vi "CRYInit Curve Library.vi"   [LabVIEW 2013]
uses:
  CRYSystem/Typedef Control/CRYData Cluster.ctl
  CRYSystem/Typedef Control/CRYResult Cluster.ctl
  CRYSystem/Typedef Control/CRYWaveform Cluster.ctl
  Global/CRYCurve Library Global.vi
  CRYMainGlobal.vi
  <vilib>/picture/picture.llb/imagedata.ctl
panel:
  # "Initialize Curve Library global variable"
types:
  T1 = cluster{"Curve OrgNames":string[], "Value OrgNames":string[], "Result OrgNames":string[], "WFM OrgNames":string[], "Curve NewNames":string[], "Value NewNames":string[], "Result NewNames":string[], "WFM NewNames":string[]}
  T2 = typedef "CRYWaveform Cluster.ctl" = cluster{"Waveform":cluster{"X0":dbl, "dX":dbl, "Y":sgl[]}, "X data":u16, "Y data":u16, "Y axis":u16, "X unit":string, "Y unit":string, "Y dB ref":dbl, "display Y":bool, "display X":bool, "Overload?":bool, "Test Info":string, "Step No.":i32, "Name":string, "protected":bool, "Sqc history":string[], "Signal Channel ID":i32, "Plot Settings":cluster{"Color":u32, "Interpolation":u8, "Point Style":u8, "Line Style":u8, "Point Color":u32, "Line Width":u8, "Bar Plot Style":u8, "Fill To":i16}, "AutoProtect":bool}
  T3 = typedef "CRYResult Cluster.ctl" = cluster{"Name":string, "Margin":dbl, "unit":string, "Verdict":bool, "Limit":string, "Max/Min":string, "protected":bool, "Step No.":i32, "Test Info":string, "AutoProtect":bool}
  T4 = cluster{"Type Name":string, "Data Name":string, "Probe VIRef Number":i32, "Probe VIRef":refnum<vi>}[]
  T5 = typedef "imagedata.ctl" = cluster{"image type":i32, "image depth":i32, "image":u8[], "mask":u8[], "colors":u32[], "Rectangle":cluster{"left":i16, "top":i16, "right":i16, "bottom":i16}}
  T6 = cluster{"Left Cell String":string, "Child Text":string[], "Child Tag":string, "Item Indent":i32, "Child Only?":bool, "Glyph Index":i32}[]
  T7 = typedef "CRYData Cluster.ctl" = cluster{"Name":string, "Curve":cluster{"x":dbl, "y":dbl, "z":dbl}[], "X data":u16, "Y data":u16, "Z data":u16, "X axis":u16, "Y axis":u16, "Z axis":u16, "X unit":string, "Y unit":string, "Z unit":string, "X dB ref":dbl, "Y dB ref":dbl, "Z dB ref":dbl, "single val":bool, "protected":bool, "display X":bool, "display Y":bool, "display Z":bool, "Test Info":string, "Step No.":i32, "Plot Settings":cluster{"Color":u32, "Interpolation":u8, "Point Style":u8, "Line Style":u8, "Point Color":u32, "Line Width":u8, "Bar Plot Style":u8, "Fill To":i16}, "AutoProtect":bool}
  T8 = typedef "CRYImageData.ctl" = cluster{"image type":i32, "image depth":i32, "image":u8[], "mask":u8[], "colors":u32[], "Rectangle":cluster{"left":i16, "top":i16, "right":i16, "bottom":i16}}
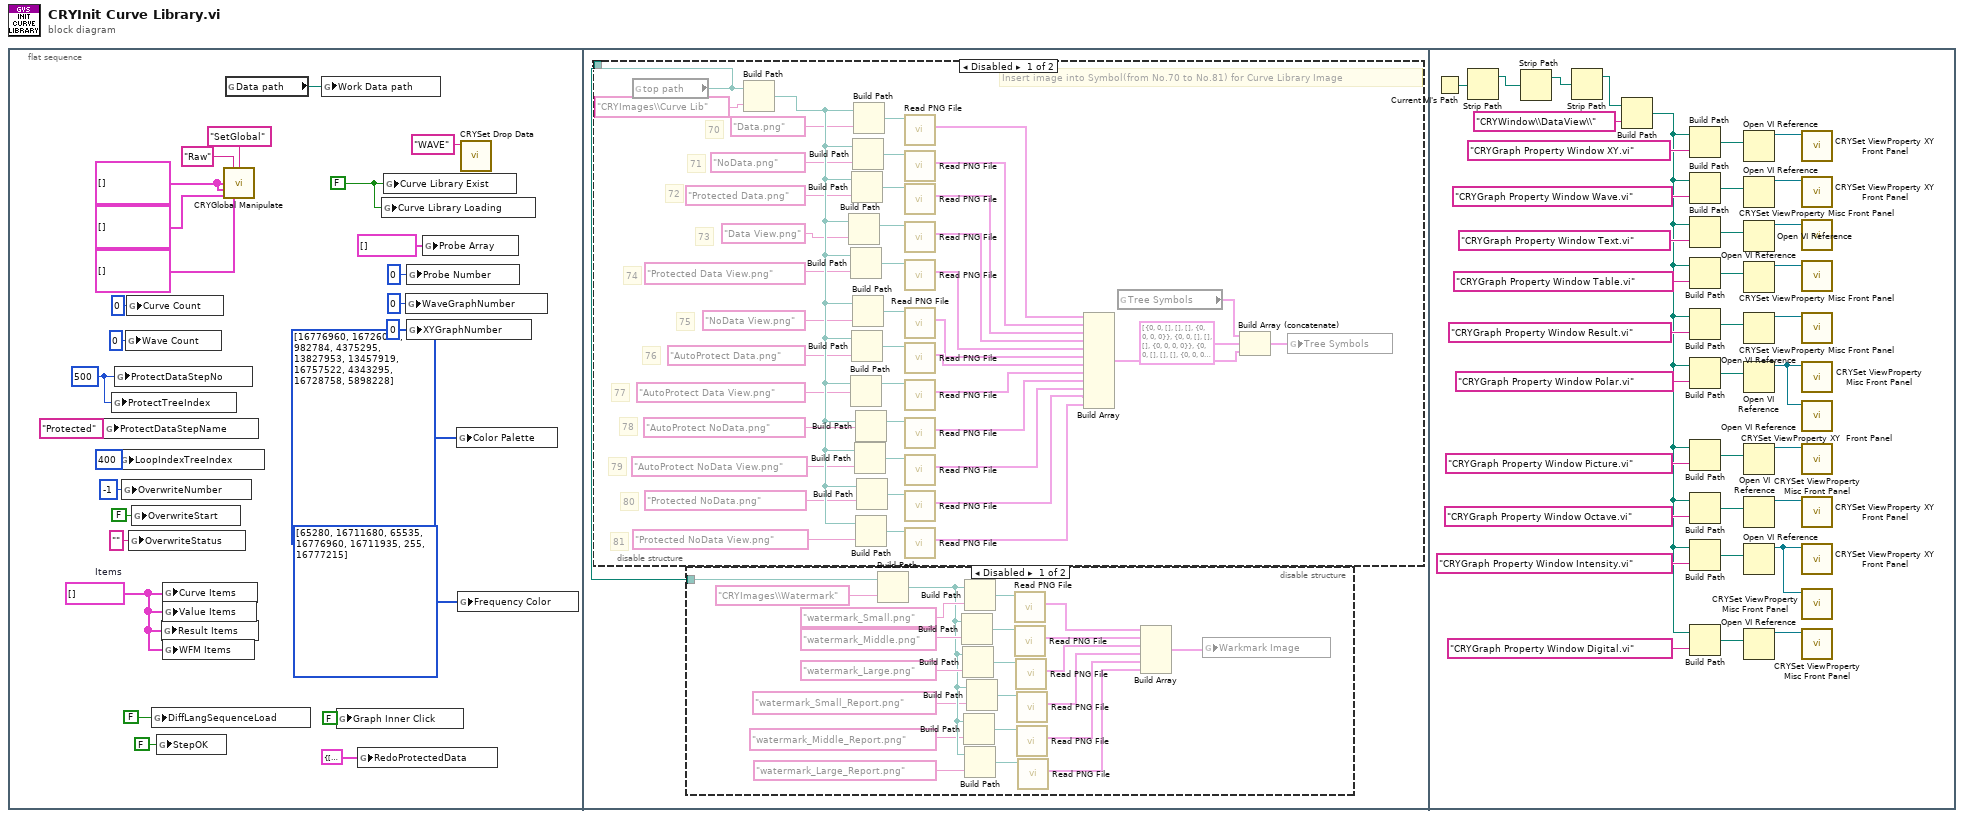
[diagram p0: block diagram]
diagram:
  n1 = flat-sequence {
    frame #0 {
      w6 = 500 ("ProtectStepNo")
      w11 = T6 []  # Items
      w14 = T7[] [] ("Curves")
      w25 = FALSE ("Exist")
      n2 = global write "CRYCurve Library Global.vi" "ProtectDataStepName"("Protected" ("ProtectDataStepName")) -> ()
      n3 = global write "CRYCurve Library Global.vi" "ProtectTreeIndex"(w6) -> ()
      n4 = global write "CRYCurve Library Global.vi" "ProtectDataStepNo"(w6) -> ()
      n5 = global write "CRYCurve Library Global.vi" "LoopIndexTreeIndex"(400 ("ProtectStepNo")) -> ()
      n6 = global write "CRYCurve Library Global.vi" "OverwriteNumber"(-1 ("ProtectStepNo")) -> ()
      n7 = global write "CRYCurve Library Global.vi" "Wave Count"(0 ("Curve Count")) -> ()
      n8 = global write "CRYCurve Library Global.vi" "Curve Count"(0 ("Curve Count")) -> ()
      n9 = global write "CRYCurve Library Global.vi" "OverwriteStatus"("" ("OverwriteStatus")) -> ()
      n10 = global write "CRYCurve Library Global.vi" "OverwriteStart"(FALSE ("OverwriteStart")) -> ()
      n11 = global write "CRYCurve Library Global.vi" "DiffLangSequenceLoad"(FALSE ("SequenceLoad")) -> ()
      n12 = global write "CRYCurve Library Global.vi" "StepOK"(FALSE ("StepOK")) -> ()
      n13 = global write "CRYCurve Library Global.vi" "Result Items"(w11) -> ()
      n14 = global write "CRYCurve Library Global.vi" "Curve Items"(w11) -> ()
      n15 = global write "CRYCurve Library Global.vi" "Value Items"(w11) -> ()
      n16 = global write "CRYCurve Library Global.vi" "WFM Items"(w11) -> ()
      n17 = call "CRYGlobal Manipulate.vi"("sOption"="Raw", "sAction"="SetGlobal", "Curves"=w14, "Values"=w14, "Results"=T3[] [], "WFM"=T2[] []) -> ()  [unwired: 3 in, 7 out]
      n18 = global read "CRYMainGlobal.vi" "Data path"() -> (w2:path)
      n19 = global write "CRYCurve Library Global.vi" "Work Data path"(w2) -> ()
      n20 = global write "CRYCurve Library Global.vi" "Graph Inner Click"(FALSE ("Graph Inner Click")) -> ()
      n21 = global write "CRYCurve Library Global.vi" "RedoProtectedData"(T1 {"Curve OrgNames"=[], "Value OrgNames"=[], "Result OrgNames"=[], "WFM OrgNames"=[], "Curve NewNames"=[], "Value NewNames"=[], "Result NewNames"=[], "WFM NewNames"=[]} ("RedoProtectedData")) -> ()
      n22 = global write "CRYCurve Library Global.vi" "Curve Library Loading"(w25) -> ()
      n23 = global write "CRYCurve Library Global.vi" "Curve Library Exist"(w25) -> ()
      n24 = global write "CRYCurve Library Global.vi" "WaveGraphNumber"(u32 0 ("WaveGraphNumber")) -> ()
      n25 = global write "CRYCurve Library Global.vi" "Probe Number"(0 ("Probe Number")) -> ()
      n26 = global write "CRYCurve Library Global.vi" "XYGraphNumber"(u32 0 ("WaveGraphNumber")) -> ()
      n27 = global write "CRYCurve Library Global.vi" "Probe Array"(T4 [] ("Probe Array")) -> ()
      n28 = global write "CRYCurve Library Global.vi" "Color Palette"(u32[] [16776960, 16726034, 982784, 4375295, 13827953, 13457919, 16757522, 4343295, 16728758, 5898228] ("Color Palette")) -> ()
      n29 = global write "CRYCurve Library Global.vi" "Frequency Color"(u32[] [65280, 16711680, 65535, 16776960, 16711935, 255, 16777215] ("Color Palette")) -> ()
      n30 = call "CRYSet Drop Data.vi"("Graph Type In"="WAVE" ("DataType In")) -> ()  [unwired: 11 out]
    }
    frame #1 {
      n31 = disable-structure shown="Disabled" {
        disable-tunnel: [w29 _] -> w28
        frame Disabled {
          # "Insert image into Symbol(from No.70 to No.81) for Curve Library Image"
          # "80"
          # "79"
          # "78"
          # "81"
          # "77"
          # "76"
          # "75"
          # "74"
          # "73"
          # "72"
          # "71"
          # "70"
          n32 = global read "CRYMainGlobal.vi" "top path"() -> (w29:path)
          n33 = Build Path(base path=w29, name or relative path="CRYImages\\Curve Lib") -> (appended path=w70:path)
          n34 = Build Path(base path=w70, name or relative path="Data View.png") -> (appended path=w35:path)
          n35 = Build Path(base path=w70, name or relative path="Protected Data View.png") -> (appended path=w34:path)
          n36 = Build Path(base path=w70, name or relative path="AutoProtect Data View.png") -> (appended path=w42:path)
          n37 = Build Path(base path=w70, name or relative path="Protected Data.png") -> (appended path=w36:path)
          n38 = Build Path(base path=w70, name or relative path="AutoProtect Data.png") -> (appended path=w41:path)
          n39 = Build Path(base path=w70, name or relative path="NoData.png") -> (appended path=w37:path)
          n40 = Build Path(base path=w70, name or relative path="NoData View.png") -> (appended path=w30:path)
          n41 = Build Path(base path=w70, name or relative path="Data.png") -> (appended path=w39:path)
          n42 = Build Path(base path=w70, name or relative path="AutoProtect NoData View.png") -> (appended path=w45:path)
          n43 = Build Path(base path=w70, name or relative path="AutoProtect NoData.png") -> (appended path=w46:path)
          n44 = Build Path(base path=w70, name or relative path="Protected NoData View.png") -> (appended path=w54:path)
          n45 = Build Path(base path=w70, name or relative path="Protected NoData.png") -> (appended path=w53:path)
          n46 = call <vilib>:"Read PNG File.vi"("path to PNG file"=w39) -> ("image data"=w56:T5)  [unwired: 1 in, 9 out]
          n47 = call <vilib>:"Read PNG File.vi"("path to PNG file"=w37) -> ("image data"=w57:T5)  [unwired: 1 in, 9 out]
          n48 = call <vilib>:"Read PNG File.vi"("path to PNG file"=w36) -> ("image data"=w58:T5)  [unwired: 1 in, 9 out]
          n49 = call <vilib>:"Read PNG File.vi"("path to PNG file"=w35) -> ("image data"=w59:T5)  [unwired: 1 in, 9 out]
          n50 = call <vilib>:"Read PNG File.vi"("path to PNG file"=w34) -> ("image data"=w60:T5)  [unwired: 1 in, 9 out]
          n51 = call <vilib>:"Read PNG File.vi"("path to PNG file"=w30) -> ("image data"=w61:T5)  [unwired: 1 in, 9 out]
          n52 = call <vilib>:"Read PNG File.vi"("path to PNG file"=w41) -> ("image data"=w62:T5)  [unwired: 1 in, 9 out]
          n53 = call <vilib>:"Read PNG File.vi"("path to PNG file"=w42) -> ("image data"=w63:T5)  [unwired: 1 in, 9 out]
          n54 = call <vilib>:"Read PNG File.vi"("path to PNG file"=w46) -> ("image data"=w64:T5)  [unwired: 1 in, 9 out]
          n55 = call <vilib>:"Read PNG File.vi"("path to PNG file"=w45) -> ("image data"=w65:T5)  [unwired: 1 in, 9 out]
          n56 = call <vilib>:"Read PNG File.vi"("path to PNG file"=w53) -> ("image data"=w66:T5)  [unwired: 1 in, 9 out]
          n57 = call <vilib>:"Read PNG File.vi"("path to PNG file"=w54) -> ("image data"=w67:T5)  [unwired: 1 in, 9 out]
          n58 = Build Array(w56, w57, w58, w59, w60, w61, w62, w63, w64, w65, w66, w67) -> (w68:T5[])
          n59 = global read "CRYMainGlobal.vi" "Tree Symbols"() -> (w55:T8[])
          n60 = Build Array (concatenate)(w55, T5[] [{"image type"=0, "image depth"=0, "image"=[], "mask"=[], "colors"=[], "Rectangle"={"left"=0, "top"=0, "right"=0, "bottom"=0}}, {"image type"=0, "image depth"=0, "image"=[], "mask"=[], "colors"=[], "Rectangle"={"left"=0, "top"=0, "right"=0, "bottom"=0}}, {"image type"=0, "image depth"=0, "image"=[], "mask"=[], "colors"=[], "Rectangle"={"left"=0, "top"=0, "right"=0, "bottom"=0}}, {"image type"=0, "image depth"=0, "image"=[], "mask"=[], "colors"=[], "Rectangle"={"left"=0, "top"=0, "right"=0, "bottom"=0}}, {"image type"=0, "image depth"=0, "image"=[], "mask"=[], "colors"=[], "Rectangle"={"left"=0, "top"=0, "right"=0, "bottom"=0}}, {"image type"=0, "image depth"=0, "image"=[], "mask"=[], "colors"=[], "Rectangle"={"left"=0, "top"=0, "right"=0, "bottom"=0}}, {"image type"=0, "image depth"=0, "image"=[], "mask"=[], "colors"=[], "Rectangle"={"left"=0, "top"=0, "right"=0, "bottom"=0}}, {"image type"=0, "image depth"=0, "image"=[], "mask"=[], "colors"=[], "Rectangle"={"left"=0, "top"=0, "right"=0, "bottom"=0}}, {"image type"=0, "image depth"=0, "image"=[], "mask"=[], "colors"=[], "Rectangle"={"left"=0, "top"=0, "right"=0, "bottom"=0}}, {"image type"=0, "image depth"=0, "image"=[], "mask"=[], "colors"=[], "Rectangle"={"left"=0, "top"=0, "right"=0, "bottom"=0}}, {"image type"=0, "image depth"=0, "image"=[], "mask"=[], "colors"=[], "Rectangle"={"left"=0, "top"=0, "right"=0, "bottom"=0}}, {"image type"=0, "image depth"=0, "image"=[], "mask"=[], "colors"=[], "Rectangle"={"left"=0, "top"=0, "right"=0, "bottom"=0}}] ("Array"), w68) -> (w71:T5[])
          n61 = global write "CRYMainGlobal.vi" "Tree Symbols"(w71) -> ()
        }
        frame Enabled {
        }
      }
      n62 = disable-structure shown="Disabled" {
        disable-tunnel: w28 -> [w93 _]
        frame Disabled {
          n63 = Build Path(base path=w93, name or relative path="CRYImages\\Watermark") -> (appended path=w79:path)
          n64 = Build Path(base path=w79, name or relative path="watermark_Middle.png") -> (appended path=w87:path)
          n65 = Build Path(base path=w79, name or relative path="watermark_Large.png") -> (appended path=w86:path)
          n66 = Build Path(base path=w79, name or relative path="watermark_Middle_Report.png") -> (appended path=w80:path)
          n67 = Build Path(base path=w79, name or relative path="watermark_Small.png") -> (appended path=w91:path)
          n68 = Build Path(base path=w79, name or relative path="watermark_Large_Report.png") -> (appended path=w81:path)
          n69 = Build Path(base path=w79, name or relative path="watermark_Small_Report.png") -> (appended path=w78:path)
          n70 = call <vilib>:"Read PNG File.vi"("path to PNG file"=w91) -> ("image data"=w90:T5)  [unwired: 8 in, 2 out]
          n71 = call <vilib>:"Read PNG File.vi"("path to PNG file"=w87) -> ("image data"=w85:T5)  [unwired: 8 in, 2 out]
          n72 = call <vilib>:"Read PNG File.vi"("path to PNG file"=w86) -> ("image data"=w84:T5)  [unwired: 8 in, 2 out]
          n73 = call <vilib>:"Read PNG File.vi"("path to PNG file"=w78) -> ("image data"=w77:T5)  [unwired: 8 in, 2 out]
          n74 = call <vilib>:"Read PNG File.vi"("path to PNG file"=w80) -> ("image data"=w76:T5)  [unwired: 8 in, 2 out]
          n75 = call <vilib>:"Read PNG File.vi"("path to PNG file"=w81) -> ("image data"=w75:T5)  [unwired: 8 in, 2 out]
          n76 = Build Array(w90, w85, w84, w77, w76, w75) -> (w89:T5[])
          n77 = global write "CRYCurve Library Global.vi" "Warkmark Image"(w89) -> ()
        }
        frame Enabled {
        }
      }
    }
    frame #2 {
      n78 = Current VI's Path() -> (path=w97:path)
      n79 = Strip Path(path=w97) -> (stripped path=w96:path)  [unwired: 1 out]
      n80 = Strip Path(path=w96) -> (stripped path=w95:path)  [unwired: 1 out]
      n81 = Strip Path(path=w95) -> (stripped path=w94:path)  [unwired: 1 out]
      n82 = Build Path(base path=w94, name or relative path="CRYWindow\\DataView\\") -> (appended path=w116:path)
      n83 = Build Path(base path=w116, name or relative path="CRYGraph Property Window XY.vi") -> (appended path=w126:path)
      n84 = Build Path(base path=w116, name or relative path="CRYGraph Property Window Wave.vi") -> (appended path=w114:path)
      n85 = Build Path(base path=w116, name or relative path="CRYGraph Property Window Text.vi") -> (appended path=w115:path)
      n86 = Build Path(base path=w116, name or relative path="CRYGraph Property Window Table.vi") -> (appended path=w112:path)
      n87 = Build Path(base path=w116, name or relative path="CRYGraph Property Window Result.vi") -> (appended path=w111:path)
      n88 = Build Path(base path=w116, name or relative path="CRYGraph Property Window Polar.vi") -> (appended path=w110:path)
      n89 = Build Path(base path=w116, name or relative path="CRYGraph Property Window Picture.vi") -> (appended path=w109:path)
      n90 = Build Path(base path=w116, name or relative path="CRYGraph Property Window Octave.vi") -> (appended path=w108:path)
      n91 = Build Path(base path=w116, name or relative path="CRYGraph Property Window Intensity.vi") -> (appended path=w106:path)
      n92 = Build Path(base path=w116, name or relative path="CRYGraph Property Window Digital.vi") -> (appended path=w105:path)
      n93 = Open VI Reference(vi path=w126) -> (vi reference=w128:refnum<vi>)  [unwired: 5 in, 1 out]
      n94 = Open VI Reference(vi path=w114) -> (vi reference=w113:refnum<vi>)  [unwired: 5 in, 1 out]
      n95 = Open VI Reference(vi path=w115) -> (vi reference=w104:refnum<vi>)  [unwired: 5 in, 1 out]
      n96 = Open VI Reference(vi path=w112) -> (vi reference=w103:refnum<vi>)  [unwired: 5 in, 1 out]
      n97 = Open VI Reference(vi path=w111) -> (vi reference=w102:refnum<vi>)  [unwired: 5 in, 1 out]
      n98 = Open VI Reference(vi path=w110) -> (vi reference=w98:refnum<vi>)  [unwired: 5 in, 1 out]
      n99 = Open VI Reference(vi path=w109) -> (vi reference=w101:refnum<vi>)  [unwired: 5 in, 1 out]
      n100 = Open VI Reference(vi path=w108) -> (vi reference=w107:refnum<vi>)  [unwired: 5 in, 1 out]
      n101 = Open VI Reference(vi path=w106) -> (vi reference=w100:refnum<vi>)  [unwired: 5 in, 1 out]
      n102 = Open VI Reference(vi path=w105) -> (vi reference=w99:refnum<vi>)  [unwired: 5 in, 1 out]
      n103 = call "CRYSet ViewProperty XY  Front Panel.vi"("Vi Ref"=w128) -> ()  [unwired: 11 in]
      n104 = call "CRYSet ViewProperty XY  Front Panel.vi"("Vi Ref"=w113) -> ()  [unwired: 11 in]
      n105 = call "CRYSet ViewProperty Misc Front Panel.vi"("Vi Ref"=w104) -> ()  [unwired: 11 in]
      n106 = call "CRYSet ViewProperty Misc Front Panel.vi"("Vi Ref"=w103) -> ()  [unwired: 11 in]
      n107 = call "CRYSet ViewProperty Misc Front Panel.vi"("Vi Ref"=w102) -> ()  [unwired: 11 in]
      n108 = call "CRYSet ViewProperty Misc Front Panel.vi"("Vi Ref"=w98) -> ()  [unwired: 11 in]
      n109 = call "CRYSet ViewProperty XY  Front Panel.vi"("Vi Ref"=w98) -> ()  [unwired: 11 in]
      n110 = call "CRYSet ViewProperty Misc Front Panel.vi"("Vi Ref"=w101) -> ()  [unwired: 11 in]
      n111 = call "CRYSet ViewProperty XY  Front Panel.vi"("Vi Ref"=w107) -> ()  [unwired: 11 in]
      n112 = call "CRYSet ViewProperty XY  Front Panel.vi"("Vi Ref"=w100) -> ()  [unwired: 11 in]
      n113 = call "CRYSet ViewProperty Misc Front Panel.vi"("Vi Ref"=w100) -> ()  [unwired: 11 in]
      n114 = call "CRYSet ViewProperty Misc Front Panel.vi"("Vi Ref"=w99) -> ()  [unwired: 11 in]
    }
  }
